vi "Delay over UDP(Tx).vi"(3 "local port(Rx)":u16=54322, 4 "remote port":u16=54322, 5 "remote IP Address":string="localhost", 6 "Iteration":i32=10) -> (0 "Array 2":cluster{"ID":string, "Timestamp":u32}[](array[cluster]), 1 "Array":cluster{"ID":string, "Timestamp":u32}[](array[cluster]), 2 "Output":i32[](array[numeric]))   [LabVIEW 2014]
uses:
  <vilib>/Utility/tdmsutil.llb/TDMS Generate Random Data (U8).vi
panel:
  out "data":u8[](array[numeric])
  out "error out(RX)":errorcluster
  out "error out(TX)":errorcluster
  in  "local port(Tx)":u16=54321
  out "possibility":i32
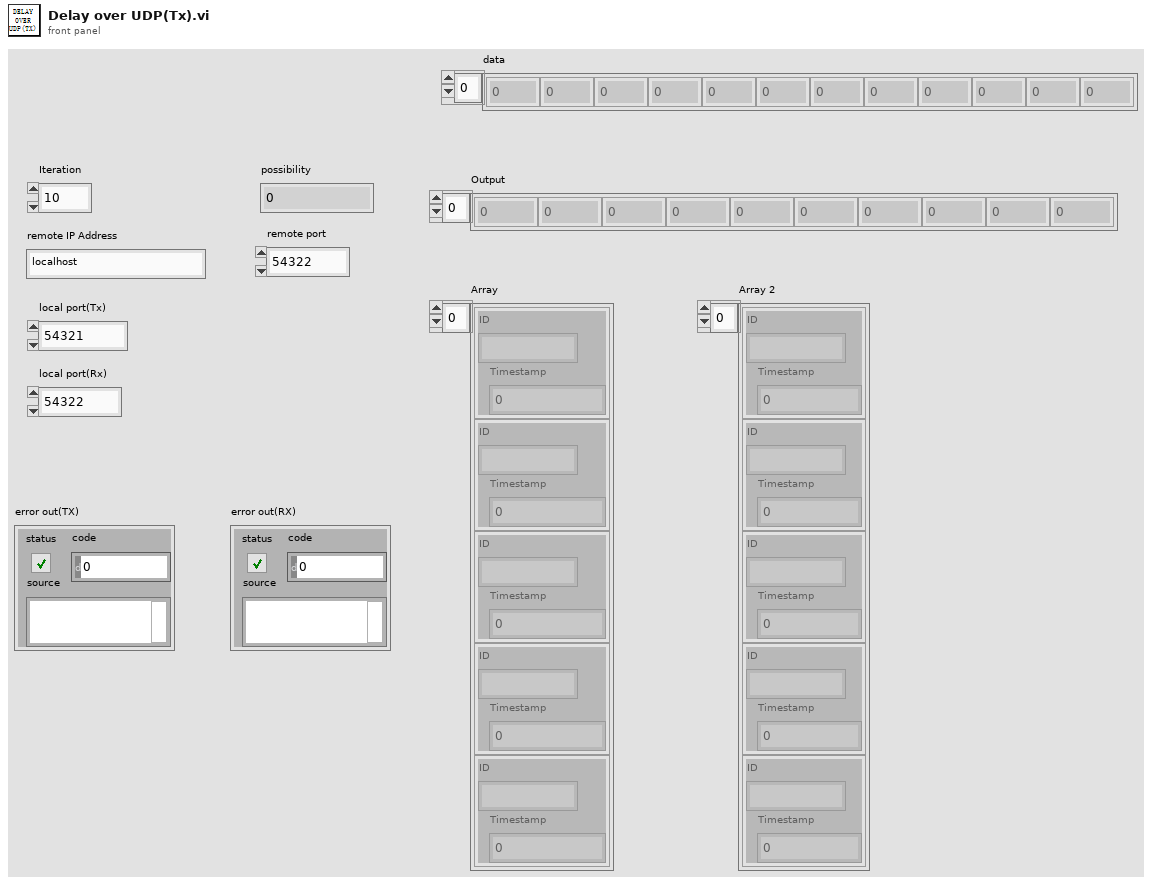
[diagram p1: front panel]
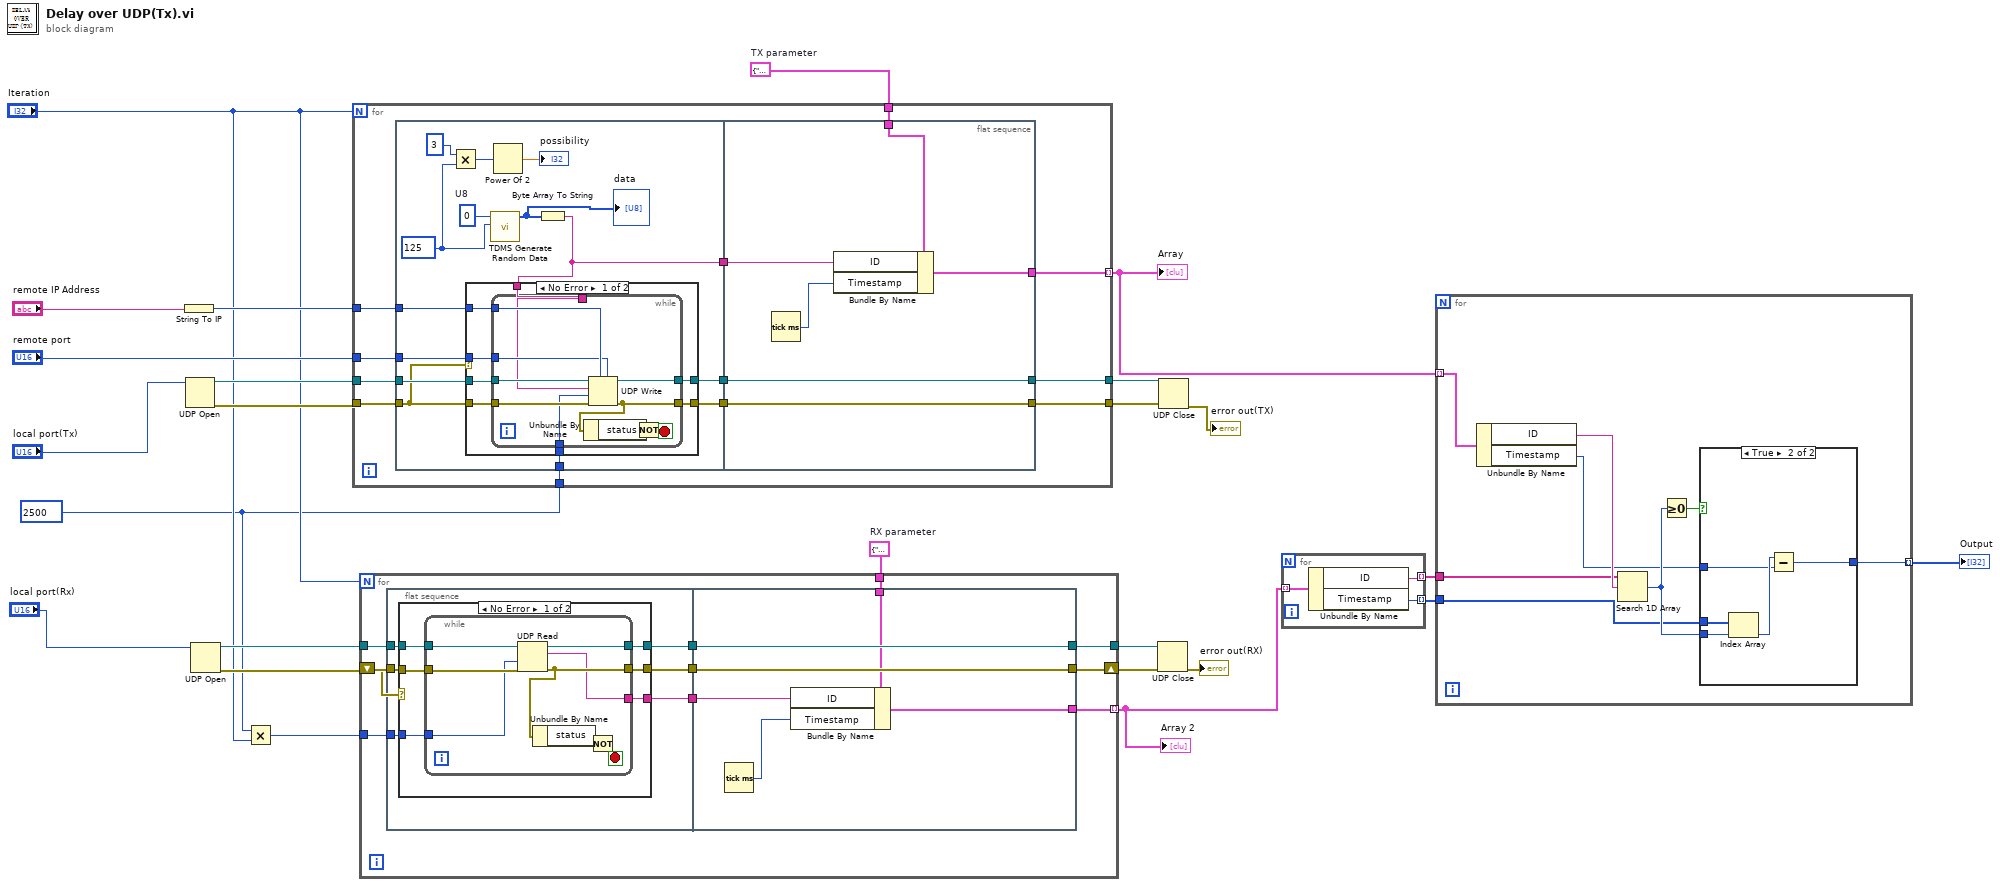
[diagram p0: block diagram]
diagram:
  w2 = 2500 ("timeout ms (25000)")
  w11 = cluster{"ID":string, "Timestamp":u32} {"ID"="string", "Timestamp"=0}  # RX parameter
  w16 = cluster{"ID":string, "Timestamp":u32} {"ID"="string", "Timestamp"=0}  # TX parameter
  n1 = String To IP(1:"remote IP Address") -> (0:w23:u32)
  n2 = UDP Open(11:"local port(Tx)") -> (port=w20:refnum<k16>, 0:w25:errorcluster)  [unwired: 4 in, 1 out]
  n3 = UDP Open(11:"local port(Rx)") -> (port=w15:refnum<k16>, 0:w14:errorcluster)  [unwired: 4 in, 1 out]
  n4 = Multiply(x=w2, y="Iteration") -> (x*y=w1:i32)
  n5 = for {
    N: "Iteration" -> [_]
    tunnel: w23 -> [w36]
    tunnel: "remote port" -> [w35]
    tunnel: w20 -> [w34]
    tunnel: [w33] -> w18
    tunnel: w16 -> [w29]
    tunnel: [w27] -> w10 mode=indexing
    tunnel: w25 -> [w37]
    tunnel: [w32] -> w19
    tunnel: w2 -> [w26]
    n6 = flat-sequence {
      tunnel: w37 -> [w39]
      tunnel: w36 -> [w46]
      tunnel: w35 -> [w45]
      tunnel: w34 -> [w44]
      tunnel: [w42] -> w31
      tunnel: [w41] -> w30
      tunnel: [w40] -> w28
      tunnel: w26 -> [w38]
      tunnel: [w73] -> w32
      tunnel: [w77] -> w33
      tunnel: w31 -> [w77]
      tunnel: w30 -> [w73]
      tunnel: w29 -> [w76]
      tunnel: w28 -> [w75]
      tunnel: [w74] -> w27
      frame #0 {
        w43 = u32 125 ("number of samples")
        w51 = u8 0  # U8
        n7 = Multiply(x=u32 3, y=w43) -> (x*y=w49:u32)
        n8 = call-poly <vilib>:"TDMS Generate Random Data.vi"("number of samples"=w43, "data type"=w51) -> ("data"=w47:u8[])  [unwired: 8 in, 1 out]
        "data" <- w47
        n9 = Power Of 2(x=w49) -> (2^x=→"possibility":dbl)
        n10 = Byte Array To String(unsigned byte array=w47) -> (string=w40:string)
        n11 = case shown="No Error" w39 {
          tunnel: w39 -> [w59 w71]
          tunnel: w46 -> [w58 _]
          tunnel: w45 -> [w57 _]
          tunnel: w44 -> [w56 w70]
          tunnel: [w55 w70] -> w42
          tunnel: [w54 w71] -> w41
          tunnel: w40 -> [w53 _]
          tunnel: w38 -> [w52 _]
          frame No Error {
            n12 = while {
              tunnel: w58 -> [w68]
              tunnel: w57 -> [w67]
              tunnel: w53 -> [w64]
              tunnel: w56 -> [w66]
              tunnel: [w65] -> w55
              tunnel: w59 -> [w69]
              tunnel: [w63] -> w54
              tunnel: w52 -> [w60]
              stop <- w61 stop-if-true
              n13 = UDP Write(address=w68, port or service name=w67, connection ID=w66, data in=w64, 8:w69, 9:w60) -> (error out=w63:errorcluster, 3:w65:refnum<k16>)
              n14 = Unbundle By Name(w63) -> ("status"=w62:bool)
              n15 = Not(x=w62) -> (.not. x?=w61:bool)
            }
          }
          frame Error {
          }
        }
      }
      frame #1 {
        n16 = Tick Count (ms)() -> (millisecond timer value=w72:u32)
        n17 = Bundle By Name(cluster=w76, "ID"=w75, "Timestamp"=w72) -> (w74:cluster{"ID":string, "Timestamp":u32})
      }
    }
  }
  "Array" <- w10
  n18 = for {
    N: "Iteration" -> [_]
    tunnel: w15 -> [w87]
    tunnel: [w86] -> w13
    shift-right: [w85] -> w12
    shift-left: w14 -> [w84]
    tunnel: w11 -> [w81]
    tunnel: [w79] -> w9 mode=indexing
    tunnel: w1 -> [w78]
    n19 = flat-sequence {
      tunnel: w87 -> [w93]
      tunnel: w84 -> [w90]
      tunnel: [w92] -> w83
      tunnel: [w91] -> w82
      tunnel: [w89] -> w80
      tunnel: w78 -> [w88]
      tunnel: [w114] -> w85
      tunnel: [w115] -> w86
      tunnel: w83 -> [w115]
      tunnel: w82 -> [w114]
      tunnel: w81 -> [w113]
      tunnel: w80 -> [w112]
      tunnel: [w110] -> w79
      frame #0 {
        n20 = case shown="No Error" w90 {
          tunnel: w93 -> [w99 w108]
          tunnel: w90 -> [w98 w109]
          tunnel: [w97 w108] -> w92
          tunnel: [w96 w109] -> w91
          tunnel: [w95 _] -> w89
          tunnel: w88 -> [w94 _]
          frame No Error {
            n21 = while {
              tunnel: w98 -> [w106]
              tunnel: w99 -> [w107]
              tunnel: [w105] -> w97
              tunnel: [w104] -> w96
              tunnel: [w102] -> w95
              tunnel: w94 -> [w100]
              stop <- w101 stop-if-true
              n22 = UDP Read(connection ID=w107, timeout ms (25000)=w100, 8:w106) -> (data out=w102:string, error out=w104:errorcluster, 3:w105:refnum<k16>)  [unwired: 1 in, 2 out]
              n23 = Unbundle By Name(w104) -> ("status"=w103:bool)
              n24 = Not(x=w103) -> (.not. x?=w101:bool)
            }
          }
          frame Error {
          }
        }
      }
      frame #1 {
        n25 = Tick Count (ms)() -> (millisecond timer value=w111:u32)
        n26 = Bundle By Name(cluster=w113, "ID"=w112, "Timestamp"=w111) -> (w110:cluster{"ID":string, "Timestamp":u32})
      }
    }
  }
  "Array 2" <- w9
  n27 = UDP Close(connection ID=w13, 8:w12) -> (error out=→"error out(RX)":errorcluster)  [unwired: 1 out]
  n28 = UDP Close(connection ID=w18, 8:w19) -> (error out=→"error out(TX)":errorcluster)  [unwired: 1 out]
  n29 = for {
    tunnel: w9 -> [w118] mode=indexing
    tunnel: [w117] -> w8 mode=indexing
    tunnel: [w116] -> w7 mode=indexing
    n30 = Unbundle By Name(w118) -> ("ID"=w117:string, "Timestamp"=w116:u32)
  }
  n31 = for {
    tunnel: w10 -> [w126] mode=indexing
    tunnel: w8 -> [w124]
    tunnel: w7 -> [w121]
    tunnel: [w119] -> w6 mode=indexing
    n32 = Unbundle By Name(w126) -> ("ID"=w125:string, "Timestamp"=w120:u32)
    n33 = Search 1D Array(1D array=w124, element=w125) -> (index of element=w122:i32)  [unwired: 1 in]
    n34 = Greater Or Equal To 0?(x=w122) -> (x >= 0?=w123:bool)
    n35 = case shown="True" w123 {
      tunnel: w122 -> [_ w131]
      tunnel: w121 -> [_ w130]
      tunnel: w120 -> [_ w128]
      tunnel: [_ w127] -> w119
      frame False {
      }
      frame True {
        n36 = Index Array(array=w130, index=w131) -> (element=w129:u32)
        n37 = Subtract(x=w129, y=w128) -> (x-y=w127:u32)
      }
    }
  }
  "Output" <- w6
